vi "ControllerTest.vi"() -> ()   [LabVIEW 2013]
panel:
  out "t: Reload positions":u32
  in  "Load Positions":dbl[](array[numeric])
  out "t: Custom command":u32
  out "IP":string caption="Custom Command: Get IP"
  out "t: Close":u32
  out "t: Get postions":u32
  out "t: Check if Moving":u32
  out "t: Move":u32
  out "t: Get position":u32
  out "t: Initialise connection":u32
  out "Is Motion Done":bool
  out "Positions":i32[](array[numeric])
  out "Positions":i32[](array[numeric])
  in  "Motor":i32=4
  in  "Target Pos":i32
  out "error out":errorcluster
  in  "PicoMotor IP":string="192.168.14.151"
  # "Before move"
  # "Position Motor 1"
  # "Position Motor 2"
  # "Position Motor 3"
  # "Position Motor 4"
  # "After move"
  # "Position Motor 1"
  # "Position Motor 2"
  # "Position Motor 3"
  # "Position Motor 4"
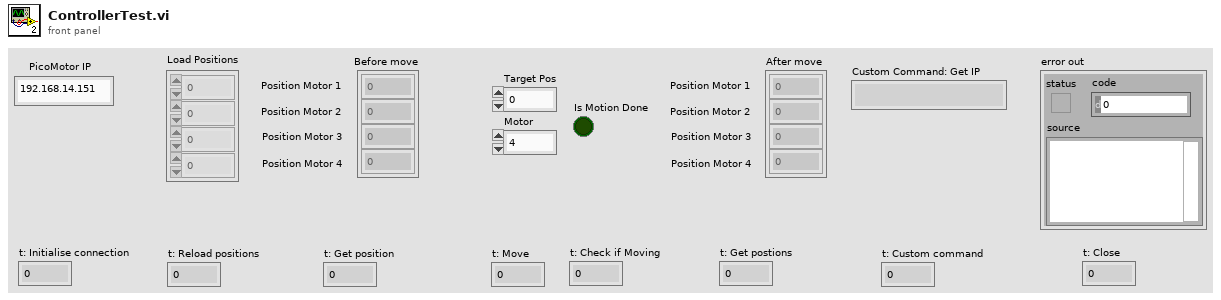
[diagram p1: front panel]
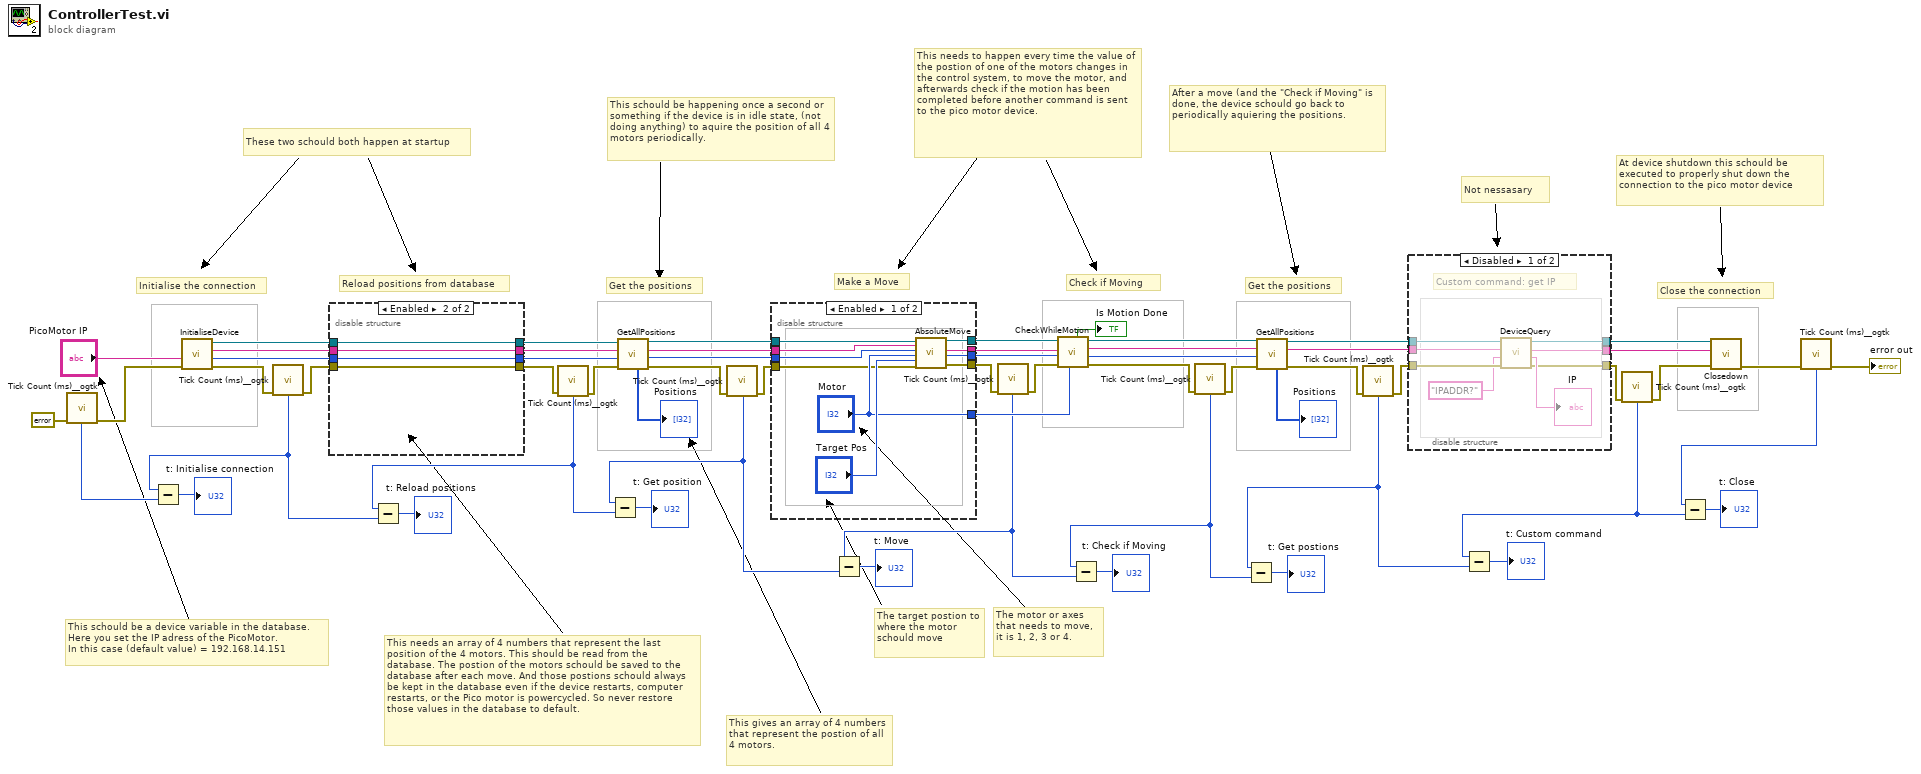
[diagram p0: block diagram]
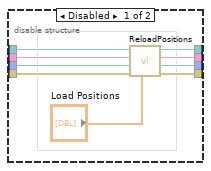
[diagram p4: hidden frame]
diagram:
  # "At device shutdown this schould be executed to properly shut down the connection to the pico motor device"
  # "After a move (and the \"Check if Moving\" is done, the device schould go back to periodically aquiering the positions."
  # "Not nessasary"
  # "This needs to happen every time the value of the postion of one of the motors changes in the control system, to move the motor, and afterwards check if the motion has been completed before another command is sent to the pico motor device."
  # "The target postion to where the motor schould move"
  # "The motor or axes that needs to move, it is 1, 2, 3 or 4."
  # "This gives an array of 4 numbers that represent the postion of all 4 motors."
  # "This schould be happening once a second or something if the device is in idle state, (not doing anything) to aquire the position of all 4 motors periodically."
  # "This needs an array of 4 numbers that represent the last position of the 4 motors. This should be read from the database. The postion of the motors schould be saved to the database after each move. And those postions schould always be kept in the database even if the device restarts, computer restarts, or the Pico motor is powercycled. So never restore those values in the database to default."
  # "These two schould both happen at startup"
  # "This schould be a device variable in the database.\nHere you set the IP adress of the PicoMotor.\nIn this case (default value) = 192.168.14.151"
  # "Reload positions from database"
  # "Check if Moving"
  # "Get the positions"
  # "Get the positions"
  # "Make a Move"
  # "Close the connection"
  # "Initialise the connection"
  n1 = call <userlib>:"Tick Count (ms)__ogtk.vi"("error in (no error)"=errorcluster {"status"=FALSE, "code"=0, "source"=""} ("error In")) -> ("error out"=w42:errorcluster, "millisecond timer value"=w46:u32)  [unwired: 9 in]
  n2 = call "InitialiseDevice.vi"("error In"=w42, "PicoMotor IP In"="PicoMotor IP") -> ("error out"=w12:errorcluster, "Device Address Out"=w7:i32, "DeviceKey Out"=w8:string, "CmdLib Out"=w11:refnum<k24>)  [unwired: 6 in]
  n3 = call <userlib>:"Tick Count (ms)__ogtk.vi"("error in (no error)"=w12) -> ("error out"=w4:errorcluster, "millisecond timer value"=w2:u32)  [unwired: 9 in]
  n4 = Subtract(x=w2, y=w46) -> (x-y=→"t: Initialise connection":u32)
  n5 = disable-structure shown="Enabled" {
    disable-tunnel: w11 -> [w68 w72]
    disable-tunnel: [w67 w72] -> w10
    disable-tunnel: [w66 w71] -> w9
    disable-tunnel: w8 -> [w65 w71]
    disable-tunnel: w7 -> [w64 w70]
    disable-tunnel: [w63 w70] -> w6
    disable-tunnel: [w62 w69] -> w5
    disable-tunnel: w4 -> [w61 w69]
    frame Disabled {
      n6 = call "ReloadPositions.vi"("Load Positions"="Load Positions", "error In"=w61, "Device Address In"=w64, "DeviceKey In"=w65, "CmdLib In"=w68) -> ("error Out"=w62:errorcluster, "Device Address Out"=w63:i32, "DeviceKey Out"=w66:string, "CmdLib Out"=w67:refnum<k24>)  [unwired: 3 in]
    }
    frame Enabled {
    }
  }
  n7 = call <userlib>:"Tick Count (ms)__ogtk.vi"("error in (no error)"=w5) -> ("error out"=w41:errorcluster, "millisecond timer value"=w1:u32)  [unwired: 9 in]
  n8 = Subtract(x=w1, y=w2) -> (x-y=→"t: Reload positions":u32)
  n9 = call "GetAllPositions.vi"("error In"=w41, "Device Address In"=w6, "DeviceKey In"=w9, "CmdLib In"=w10) -> ("error out"=w40:errorcluster, "Device Address Out"=w59:i32, "DeviceKey Out"=w57:string, "CmdLib Out"=w58:refnum<k24>, "Positions"=→"Positions":i32[])  [unwired: 3 in]
  n10 = call <userlib>:"Tick Count (ms)__ogtk.vi"("error in (no error)"=w40) -> ("error out"=w39:errorcluster, "millisecond timer value"=w27:u32)  [unwired: 9 in]
  n11 = Subtract(x=w27, y=w1) -> (x-y=→"t: Get position":u32)
  n12 = disable-structure shown="Enabled" {
    disable-tunnel: w59 -> [w81 w84]
    disable-tunnel: w58 -> [w80 w86]
    disable-tunnel: w57 -> [w79 w85]
    disable-tunnel: [w78 w86] -> w54
    disable-tunnel: [w77 w85] -> w52
    disable-tunnel: [w76 w84] -> w50
    disable-tunnel: ["Motor" _] -> w48
    disable-tunnel: w39 -> [w74 w83]
    disable-tunnel: [w73 w83] -> w38
    frame Enabled {
      n13 = call "AbsoluteMove.vi"("CmdLib In"=w80, "DeviceKey In"=w79, "Device Address In"=w81, "Motor"="Motor", "Target Pos"="Target Pos", "error in (no error)"=w74) -> ("CmdLib Out"=w78:refnum<k24>, "DeviceKey Out"=w77:string, "Device Address Out"=w76:i32, "error out"=w73:errorcluster)  [unwired: 10 in]
    }
    frame Disabled {
    }
  }
  n14 = call <userlib>:"Tick Count (ms)__ogtk.vi"("error in (no error)"=w38) -> ("error out"=w37:errorcluster, "millisecond timer value"=w26:u32)  [unwired: 9 in]
  n15 = Subtract(x=w26, y=w27) -> (x-y=→"t: Move":u32)
  n16 = call "CheckWhileMotion.vi"("Motor"=w48, "error In"=w37, "Device Address In"=w50, "DeviceKey In"=w52, "CmdLib In"=w54) -> ("error Out"=w36:errorcluster, "Device Address Out"=w49:i32, "DeviceKey Out"=w51:string, "CmdLib Out"=w53:refnum<k24>, "Is Motion Done"=→"Is Motion Done":bool)  [unwired: 2 in]
  n17 = call <userlib>:"Tick Count (ms)__ogtk.vi"("error in (no error)"=w36) -> ("error out"=w35:errorcluster, "millisecond timer value"=w25:u32)  [unwired: 9 in]
  n18 = Subtract(x=w25, y=w26) -> (x-y=→"t: Check if Moving":u32)
  n19 = call "GetAllPositions.vi"("error In"=w35, "Device Address In"=w49, "DeviceKey In"=w51, "CmdLib In"=w53) -> ("error out"=w34:errorcluster, "DeviceKey Out"=w19:string, "CmdLib Out"=w22:refnum<k24>, "Positions"=→"Positions":i32[])  [unwired: 3 in, 1 out]
  n20 = call <userlib>:"Tick Count (ms)__ogtk.vi"("error in (no error)"=w34) -> ("error out"=w21:errorcluster, "millisecond timer value"=w24:u32)  [unwired: 9 in]
  n21 = Subtract(x=w24, y=w25) -> (x-y=→"t: Get postions":u32)
  n22 = disable-structure shown="Disabled" {
    disable-tunnel: [w94 w97] -> w23
    disable-tunnel: w22 -> [w93 w97]
    disable-tunnel: w21 -> [w92 w95]
    disable-tunnel: [w91 w96] -> w20
    disable-tunnel: w19 -> [w90 w96]
    disable-tunnel: [w87 w95] -> w17
    frame Disabled {
      # "Custom command: get IP"
      n23 = call "DeviceQuery.vi"("error in (no error)"=w92, "Command"="IPADDR?", "DeviceKey In"=w90, "CmdLib In"=w93) -> ("error out"=w87:errorcluster, "Response"=→"IP":string, "DeviceKey Out"=w91:string, "CmdLib Out"=w94:refnum<k24>)
    }
    frame Enabled {
    }
  }
  n24 = call <userlib>:"Tick Count (ms)__ogtk.vi"("error in (no error)"=w17) -> ("error out"=w16:errorcluster, "millisecond timer value"=w14:u32)  [unwired: 9 in]
  n25 = Subtract(x=w14, y=w24) -> (x-y=→"t: Custom command":u32)
  n26 = call "Closedown.vi"("error In"=w16, "DeviceKey In"=w20, "CmdLib In"=w23) -> ("error out"=w28:errorcluster)  [unwired: 8 in]
  n27 = call <userlib>:"Tick Count (ms)__ogtk.vi"("error in (no error)"=w28) -> ("error out"=→"error out":errorcluster, "millisecond timer value"=w15:u32)  [unwired: 9 in]
  n28 = Subtract(x=w15, y=w14) -> (x-y=→"t: Close":u32)
